vi "Add Points to Series_DBL[].vi"(6 "YValuesPerPoint":i32=1, 8 "error in (no error)":errorcluster, 9 "Data":cluster{"X":dbl, "Y":dbl}[](array[cluster])=[{"X"=0.0, "Y"=0.25}, {"X"=1.0, "Y"=0.75}, {"X"=2.0, "Y"=1.95}, {"X"=3.0, "Y"=1.6}, {"X"=4.0, "Y"=1.6}, {"X"=5.0, "Y"=2.5}, {"X"=6.0, "Y"=1.8}, {"X"=7.0, "Y"=1.26}], 10 ".NET MSChart Series":refnum<k24>) -> (0 "error out":errorcluster)   [LabVIEW 2015, in "Graph Extensions MSChart.lvlib"]
uses:
  Graph Extensions MSChart.lvlib
  System.Windows.Forms.DataVisualization
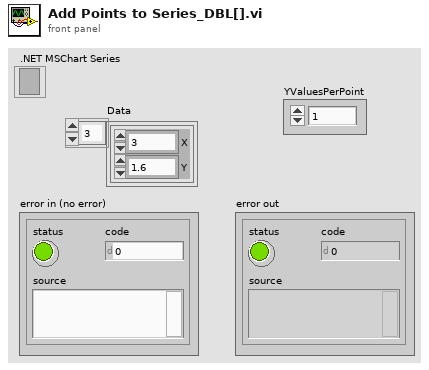
[diagram p1: front panel]
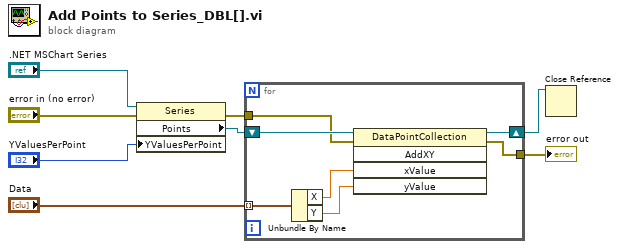
[diagram p0: block diagram]
diagram:
  n1 = property class="Series"(reference=".NET MSChart Series", error in="error in (no error)", "YValuesPerPoint"="YValuesPerPoint") -> (error out=w4:errorcluster, "Points"=w3:refnum<k24>)  [unwired: 1 out]
  n2 = for {
    tunnel: "Data" -> [w10] mode=indexing
    tunnel: [w13] -> w8
    shift-right: [w14] -> w1
    shift-left: w3 -> [w15]
    tunnel: w4 -> [w12]
    n3 = Unbundle By Name(w10) -> ("X"=w9:dbl, "Y"=w11:dbl)
    n4 = invoke class="DataPointCollection" method="AddXY"(reference=w15, error in=w12, "xValue"=w9, "yValue"=w11) -> (reference out=w14:refnum<k24>, error out=w13:errorcluster)  [unwired: 1 in, 3 out]
  }
  "error out" <- w8
  n5 = Close Reference(reference=w1) -> ()  [unwired: 1 in, 1 out]
